vi "configureAcquisition.vi"(6 "imagePaths":path[](array[path]), 7 "save?":bool, 8 "error in (no error)":errorcluster, 9 "numberImages":i32, 10 "settingsPath":path, 11 "CameraNetworkController in":refnum<class "CameraNetworkController.lvclass">) -> (0 "error out":errorcluster, 3 "CameraNetworkController out":refnum<class "CameraNetworkController.lvclass">)   [LabVIEW 2011, in "Hardware.lvlib" / "HWControllers.lvlib" / "CameraNetworkController.lvclass"]
uses:
  CameraNetworkController.lvclass
  Tools/CameraSettings/CamaraSettings.lvclass
  CameraNetworkController.lvclass/CameraNetworkController.ctl
  NetworkClient/NetworkServer.lvclass
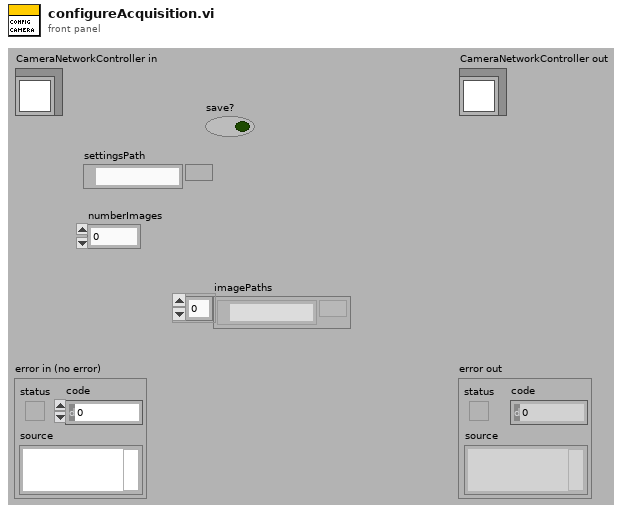
[diagram p1: front panel]
types:
  T1 = cluster{"CamaraSettings":refnum<class "CamaraSettings.lvclass">, "saveImages?":bool, "imagePaths":path[], "number of Images":i32}
  T2 = cluster{"Message":enum16{"Idle", "initialise", "configureAcquisition", "setTemperature", "getTemperature", "start", "stop", "sendImage", "close", "error", "ExitApp"}, "Data":variant}
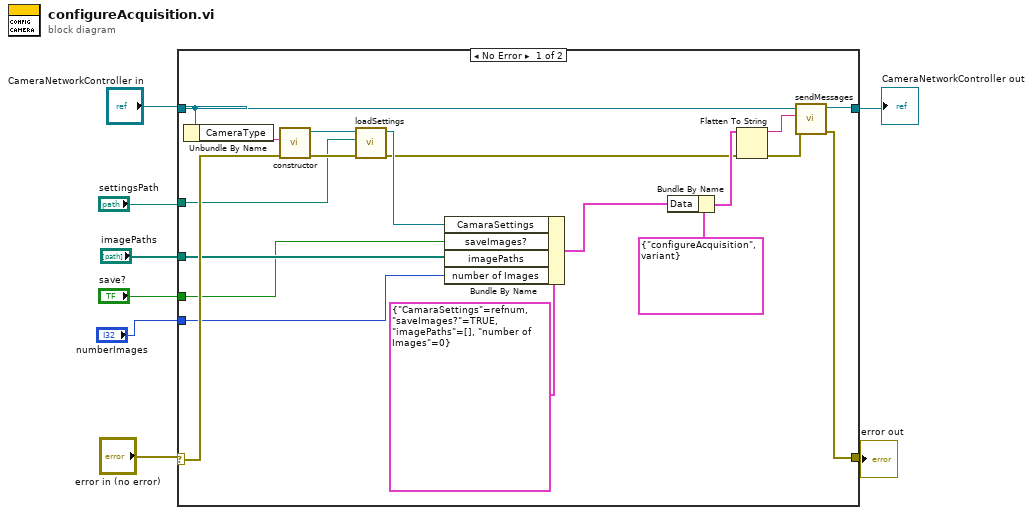
[diagram p0: block diagram]
diagram:
  n1 = case shown="No Error" "error in (no error)" {
    selector: "error in (no error)" -> [w19 w29]
    tunnel: [w22 w29] -> w6
    tunnel: [w27 w28] -> w5
    tunnel: "CameraNetworkController in" -> [w21 w28]
    tunnel: "settingsPath" -> [w16 _]
    tunnel: "numberImages" -> [w14 _]
    tunnel: "imagePaths" -> [w12 _]
    tunnel: "save?" -> [w11 _]
    frame No Error {
      n2 = Unbundle By Name(w21) -> ("CameraType"=w20:string)
      n3 = call "constructor.vi"("error in (no error)"=w19, "camera settings"=w20) -> ("error out"=w17:errorcluster, "CamaraSettings out"=w18:refnum<class "CamaraSettings.lvclass">)  [unwired: 8 in]
      n4 = call-dynamic "loadSettings.vi"("error in (no error)"=w17, "Path"=w16, "CamaraSettings in"=w18) -> ("error out"=w9:errorcluster, "CamaraSettings out"=w13:refnum<class "CamaraSettings.lvclass">)  [unwired: 7 in]
      n5 = Bundle By Name(cluster=T1 {"CamaraSettings"=refnum, "saveImages?"=TRUE, "imagePaths"=[], "number of Images"=0}, "CamaraSettings"=w13, "saveImages?"=w11, "imagePaths"=w12, "number of Images"=w14) -> (w10:T1)
      n6 = Bundle By Name(cluster=T2 {"Message"=enum."configureAcquisition", "Data"=variant}, "Data"=w10) -> (w25:T2)
      n7 = Flatten To String(anything=w25, error in (no error)=w9) -> (data string=w23:string, error out=w24:errorcluster)  [unwired: 3 out]
      n8 = call "sendMessages.vi"("error in (no error)"=w24, "messageString"=w23, "NetworkClient in"=w21) -> ("error out"=w22:errorcluster, "NetworkClient out"=w27:refnum<class "CameraNetworkController.lvclass">)  [unwired: 7 in]
    }
    frame Error {
    }
  }
  "error out" <- w6
  "CameraNetworkController out" <- w5
